vi "Teleop - Copy.vi"(10 "Match Info":T3={"Autonomous Elapsed Seconds"=0.0, "TeleOp Elapsed Seconds"=0.0, "Disabled Elapsed Seconds"=0.0, "Visited Autonomous"=FALSE, "Visited TeleOp"=FALSE, "Visited Disabled"=FALSE, "Autonomous Settings"={"Autonomous Style"=enum."Independent", "VI Refnum"=refnum}}, 11 "Call Context":T4) -> ()   [LabVIEW 2015]
doc: "This VI is called for each TeleOp packet received from the DS where the robot is not disabled. It is often used to read from the joysticks and update I/O or to update setpoints for timed control loops. It should complete and return within 20 milliseconds or it may miss DS packets."
uses:
  <vilib>/Rock Robotics/WPI/DriverStation/WPI_DriverStationDerivedRobotMode.ctl
  <vilib>/Rock Robotics/WPI/DriverStation/WPI_DriverStationMatch Info.ctl
  <vilib>/Rock Robotics/WPI/Joystick/WPI_JoystickDevRef.ctl
  <vilib>/Rock Robotics/WPI/Joystick/WPI_JoystickDeviceEnum.ctl
  <vilib>/Rock Robotics/WPI/Utilities/WPI_GetSetVariantRefNum.vi
  <vilib>/Rock Robotics/Network Tables/NT Read Boolean.vi
  <vilib>/Rock Robotics/Network Tables/NT Read Number.vi
  Robot Global Data.vi
  <vilib>/Rock Robotics/Network Tables/NT Write Numeric Array.vi
  <vilib>/Rock Robotics/Network Tables/NT Write Boolean Array.vi
  <vilib>/Rock Robotics/Network Tables/NT Write Number.vi
panel:
  in  "Intake Speed 2":dbl=-30.0 format="%#_13g"
  out "Joystick0":T1={"Device"=enum."USB 1"}
  out "Position Control":dbl
  in  "Intake Speed":dbl=-30.0 format="%#_13g"
  out "Sample Slider 0":dbl(slide) scale=0.0..5.0
  out "Sample Boolean 1":bool
  out "Sample Boolean 0":bool
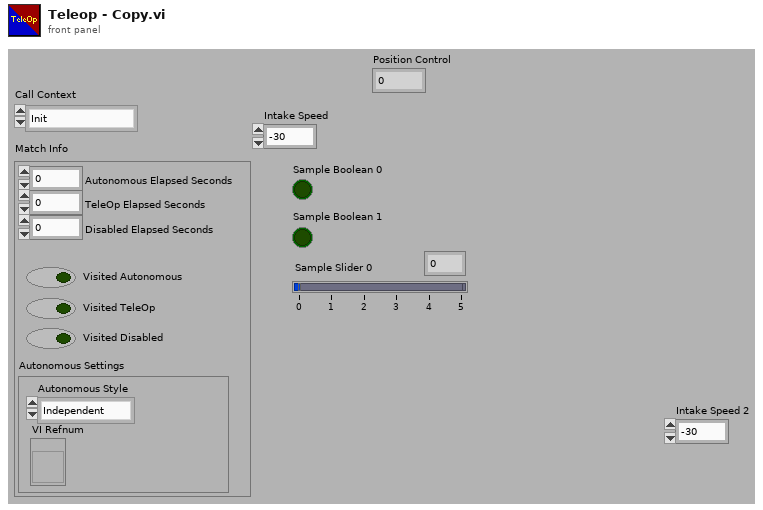
[diagram p1: front panel]
types:
  T1 = typedef "WPI_JoystickDevRef.ctl" = cluster{"Device":T2}
  T2 = typedef "WPI_JoystickDeviceEnum.ctl" = enum16{"USB 0", "USB 1", "USB 2", "USB 3", "USB 4", "USB 5"}
  T3 = typedef "WPI_DriverStationMatch Info.ctl" = cluster{"Autonomous Elapsed Seconds":dbl, "TeleOp Elapsed Seconds":dbl, "Disabled Elapsed Seconds":dbl, "Visited Autonomous":bool, "Visited TeleOp":bool, "Visited Disabled":bool, "Autonomous Settings":cluster{"Autonomous Style":enum16{"Iterative", "Independent"}, "VI Refnum":refnum<vi>}}
  T4 = typedef "WPI_DriverStationDerivedRobotMode.ctl" = enum16{"Init", "Execute", "Stop"}
  T5 = typedef "WPI_DigitalInputDevRef.ctl" = cluster{"DevStatus":errorcluster, "DIO Channel":T6}
  T6 = typedef "FPGA_DIOChannel.ctl" = enum8{"DIO 0", "DIO 1", "DIO 2", "DIO 3", "DIO 4", "DIO 5", "DIO 6", "DIO 7", "DIO 8", "DIO 9", "DIO MXP 0", "DIO MXP 1", "DIO MXP 2", "DIO MXP 3", "DIO MXP 4", "DIO MXP 5", "DIO MXP 6", "DIO MXP 7", "DIO MXP 8", "DIO MXP 9", "DIO MXP 10", "DIO MXP 11", "DIO MXP 12", "DIO MXP 13", "DIO MXP 14", "DIO MXP 15", "Invalid"}
  T7 = cluster{"LeftX":dbl, "LeftY":dbl, "LTrigger":dbl, "RTrigger":dbl, "RightX":dbl, "RightY":dbl, "RightY 2":dbl, "RightX 2":dbl}
  T8 = cluster{"ButtonA":bool, "ButtonB":bool, "ButtonX":bool, "ButtonY":bool, "ButtonLB":bool, "ButtonRB":bool, "ButtonBack":bool, "ButtonStart":bool, "Button1":bool, "Button2":bool}
  T9 = typedef "WPI_MotorControlDeviceRef.ctl" = cluster{"DeviceStatus":errorcluster, "Type":T10, "PWM":cluster{"PWM Channel":T11, "DeadBand":T12}, "CAN":cluster{"Device Number":u8, "Control Mode":T13, "Semaphore":T14, "Max Vout":dbl, "TalonSRX Control Mode":T15}, "Invert":bool}
  T10 = typedef "WPI_MotorControlType.ctl" = enum16{"PWM", "CAN", "CANTalonSRX"}
  T11 = typedef "FPGA_DIOPWMChannel.ctl" = enum8{"PWM 0", "PWM 1", "PWM 2", "PWM 3", "PWM 4", "PWM 5", "PWM 6", "PWM 7", "PWM 8", "PWM 9", "PWM MXP 0", "PWM MXP 1", "PWM MXP 2", "PWM MXP 3", "PWM MXP 4", "PWM MXP 5", "PWM MXP 6", "PWM MXP 7", "PWM MXP 8", "PWM MXP 9", "Invalid"}
  T12 = typedef "WPI_PWMDeadband.ctl" = cluster{"Name":string, "maxPositivePwm":i32, "minPositivePwm":i32, "centerPwm":i32, "maxNegativePwm":i32, "minNegativePwm":i32, "angularRange":u16}
  T13 = typedef "WPI_CANJaguar_ControlMode.ctl" = enum8{"Percent VBus", "Current", "Speed", "Position", "Voltage"}
  T14 = typedef "Semaphore RefNum" = refnum<k1>
  T15 = typedef "WPI_CANTalonSRX_APIControlMode.ctl" = enum8{"Percent VBus", "Speed", "Position", "Slave", "Unchanged / Invalid", "Voltage Compensation", "Current", "Motion Profile"}
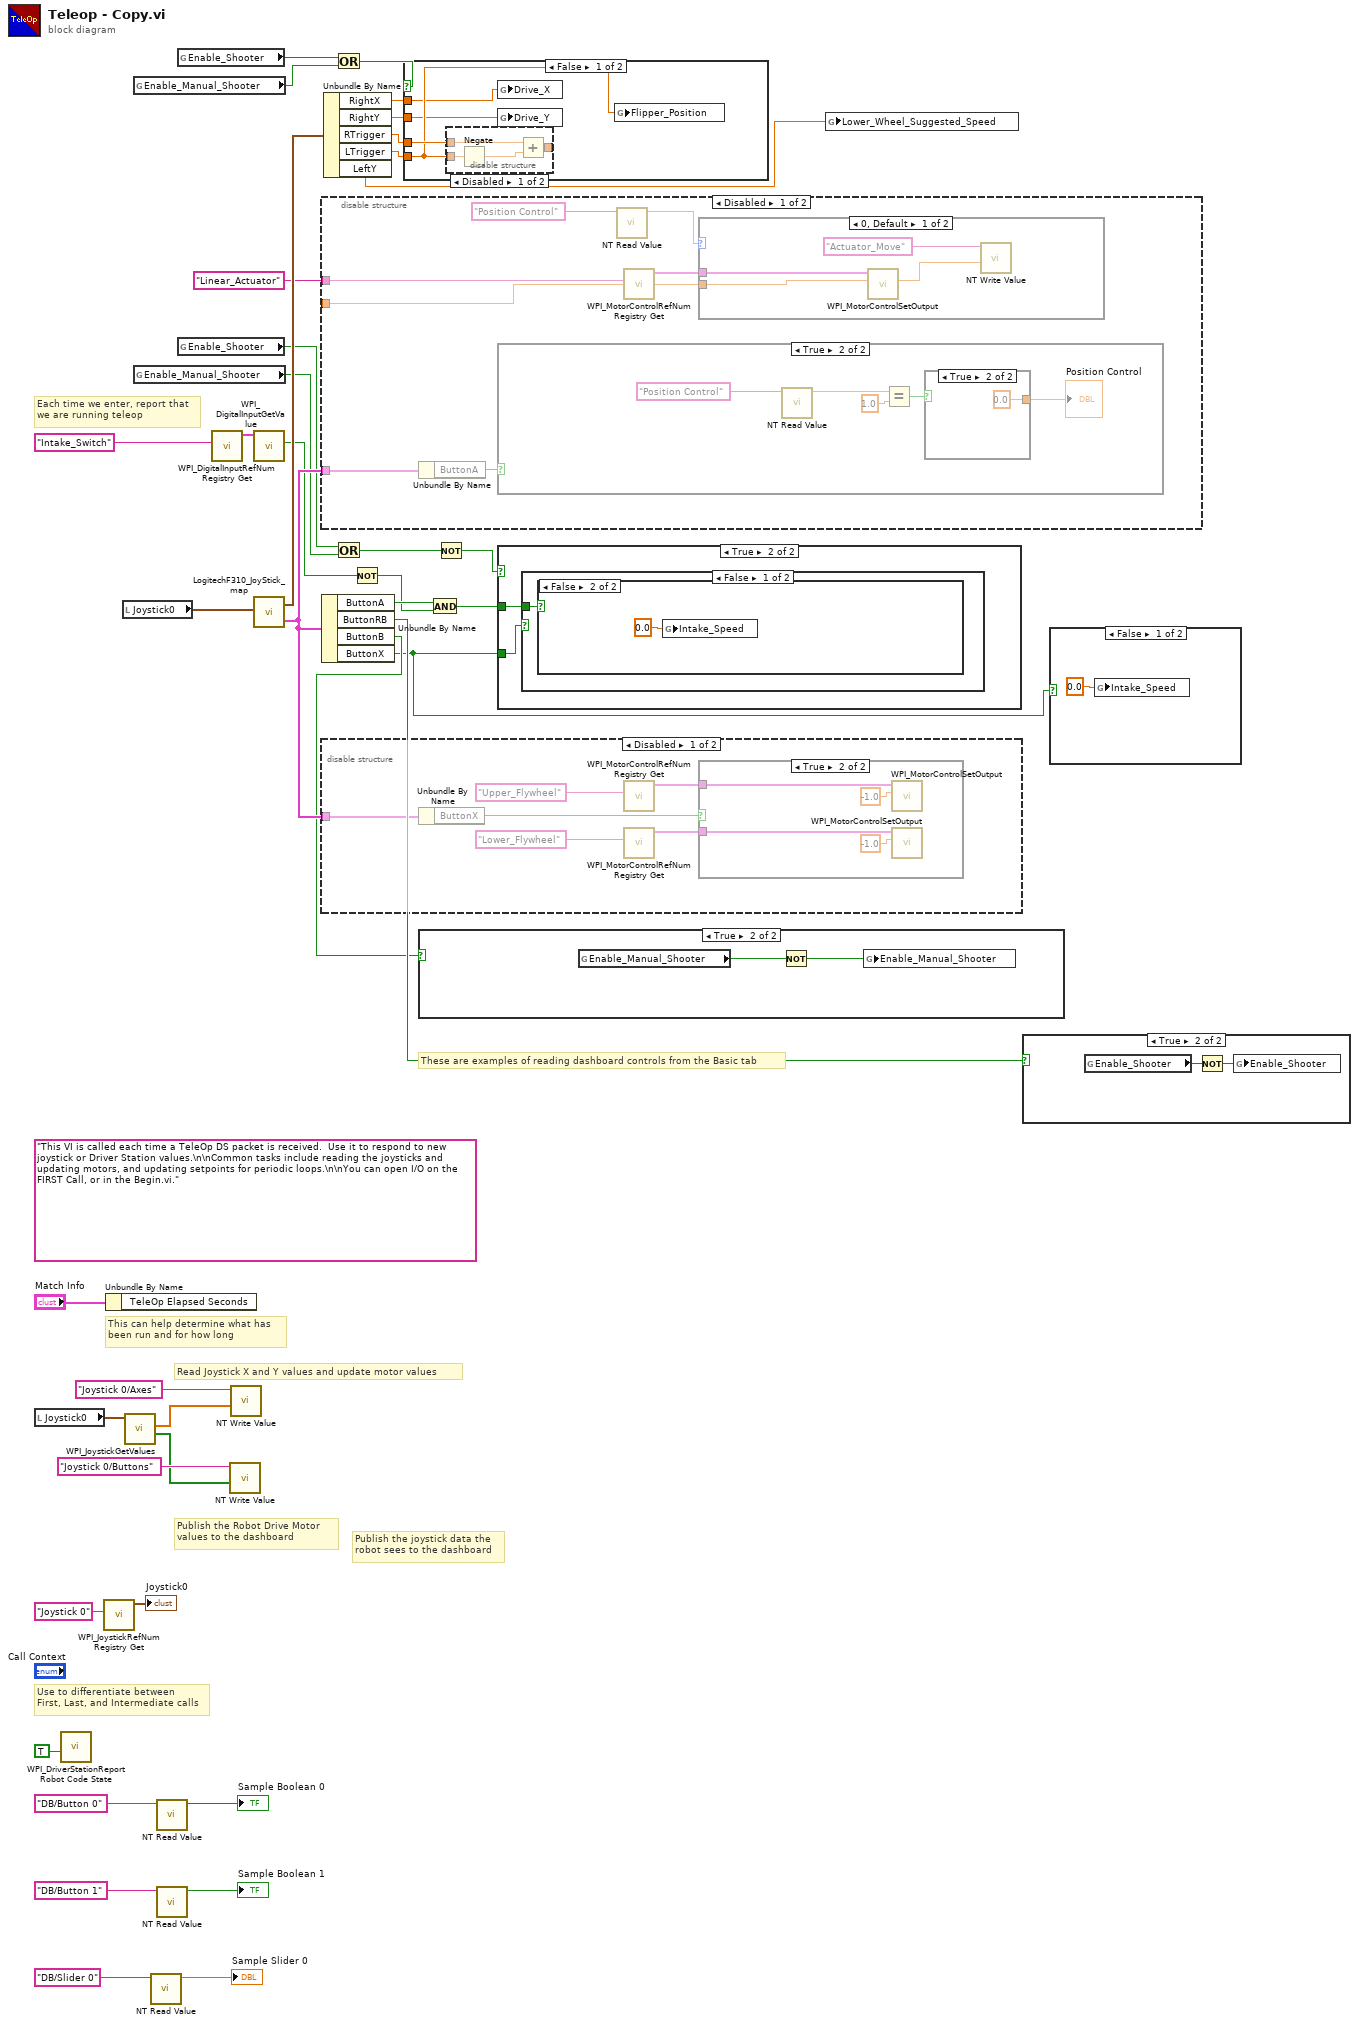
[diagram p0: block diagram]
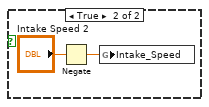
[diagram p2: hidden frame]
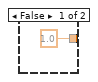
[diagram p6: hidden frame]
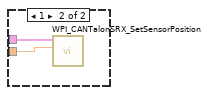
[diagram p7: hidden frame]
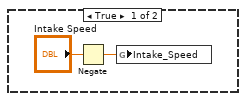
[diagram p10: hidden frame]
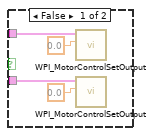
[diagram p14: hidden frame]
diagram:
  (unwired) "This VI is called each time a TeleOp DS packet is received.  Use it to respond to new joystick or Driver Station values.\n\nCommon tasks include reading the joysticks and updating motors, and updating setpoints for periodic loops.\n\nYou can open I/O on the FIRST Call, or in the Begin.vi."
  # "These are examples of reading dashboard controls from the Basic tab"
  # "Publish the Robot Drive Motor\nvalues to the dashboard"
  # "Publish the joystick data the\nrobot sees to the dashboard"
  # "Each time we enter, report that\nwe are running teleop"
  # "Use to differentiate between\nFirst, Last, and Intermediate calls"
  # "This can help determine what has\nbeen run and for how long"
  # "Read Joystick X and Y values and update motor values"
  n1 = local read "Joystick0"() -> (w8:T1)
  n2 = call <vilib>:"WPI_DriverStationReport Robot Code State.vi"("TeleOp"=TRUE ("Autonomous")) -> ()  [unwired: 10 in, 1 out]
  n3 = call <vilib>:"WPI_JoystickRefNum Registry Get.vi"("refnum name"="Joystick 0") -> ("JoystickDevRef"=→"Joystick0":T1)  [unwired: 1 in, 9 out]
  n4 = Unbundle By Name("Match Info") -> ()  [unwired: 1 out]
  n5 = local read "Joystick0"() -> (w5:T1)
  n6 = call <vilib>:"WPI_JoystickGetValues.vi"("JoystickDevRef"=w8) -> ("Buttons"=w34:bool[], "Axes"=w35:dbl[])  [unwired: 6 in, 3 out]
  n7 = global read "Robot Global Data.vi" "Enable_Manual_Shooter"() -> (w11:bool)
  n8 = global read "Robot Global Data.vi" "Enable_Manual_Shooter"() -> (w13:bool)
  n9 = call-poly <vilib>:"NT Read Value.vi"("Name"="DB/Slider 0" ("refnum name")) -> ("Numeric"=→"Sample Slider 0":dbl)  [unwired: 9 in, 1 out]
  n10 = call-poly <vilib>:"NT Read Value.vi"("Name"="DB/Button 0" ("refnum name")) -> ("Boolean"=→"Sample Boolean 0":bool)  [unwired: 9 in, 1 out]
  n11 = call-poly <vilib>:"NT Read Value.vi"("Name"="DB/Button 1" ("refnum name")) -> ("Boolean"=→"Sample Boolean 1":bool)  [unwired: 9 in, 1 out]
  n12 = global read "Robot Global Data.vi" "Enable_Shooter"() -> (w19:bool)
  n13 = global read "Robot Global Data.vi" "Enable_Shooter"() -> (w18:bool)
  n14 = call <vilib>:"WPI_DigitalInputRefNum Registry Get.vi"("refnum name"="Intake_Switch") -> ("DigitalInputDevRef"=w23:T5)  [unwired: 9 in, 1 out]
  n15 = call-poly <vilib>:"NT Write Value.vi"("Boolean Array"=w34, "Name"="Joystick 0/Buttons") -> ()  [unwired: 9 in, 1 out]
  n16 = call-poly <vilib>:"NT Write Value.vi"("Numeric Array"=w35, "Name"="Joystick 0/Axes") -> ()  [unwired: 9 in, 1 out]
  n17 = call <vilib>:"WPI_DigitalInputGetValue.vi"("DigitalInputDevRef"=w23) -> ("Value"=w3:bool)  [unwired: 8 in, 2 out]
  n18 = call "LogitechF310_JoyStick_map.vi"("JoystickDevRef"=w5) -> ("AxesCluster"=w27:T7, "ButtonsCluster"=w24:T8)
  n19 = disable-structure shown="Disabled" {
    disable-tunnel: "Linear_Actuator" ("refnum name") -> [w47 _]
    disable-tunnel: _ -> [w45 _]
    disable-tunnel: w24 -> [w44 _]
    frame Disabled {
      n20 = Unbundle By Name(w44) -> ("ButtonA"=w43:bool)
      n21 = case shown="True" w43 {
        frame False {
        }
        frame True {
          n22 = call-poly <vilib>:"NT Read Value.vi"("Name"="Position Control") -> ("Numeric"=w49:dbl)  [unwired: 9 in, 1 out]
          n23 = Equal?(x=w49, y=1.0) -> (x = y?=w51:bool)
          n24 = case shown="True" w51 {
            tunnel: [1.0 ("Position Control") 0.0 ("Position Control")] -> w48
            frame False {
            }
            frame True {
            }
          }
          "Position Control" <- w48
        }
      }
      n25 = call-poly <vilib>:"NT Read Value.vi"("Name"="Position Control") -> ("Numeric"=w41:dbl)  [unwired: 9 in, 1 out]
      n26 = call <vilib>:"WPI_MotorControlRefNum Registry Get.vi"("refnum name"=w47) -> ("MotorControlDevRef"=w46:T9)  [unwired: 9 in, 1 out]
      n27 = case shown="0, Default" w41 {
        tunnel: w46 -> [w55 w60]
        tunnel: w45 -> [w56 w59]
        frame 0, Default {
          n28 = call <vilib>:"WPI_MotorControlSetOutput.vi"("Output"=w56, "MotorControlDevRef"=w55) -> ("Motor Output"=w58:dbl)  [unwired: 7 in, 2 out]
          n29 = call-poly <vilib>:"NT Write Value.vi"("Numeric"=w58, "Name"="Actuator_Move") -> ()  [unwired: 9 in, 1 out]
        }
        frame 1 {
          n30 = call <vilib>:"WPI_CANTalonSRX_SetSensorPosition.vi"("New Sensor Position"=w59, "CAN Talon SRX Ref"=w60) -> ()  [unwired: 8 in, 2 out]
        }
      }
    }
    frame Enabled {
    }
  }
  n31 = Unbundle By Name(w24) -> ("ButtonA"=w22:bool, "ButtonRB"=w16:bool, "ButtonB"=w15:bool, "ButtonX"=w1:bool)
  n32 = disable-structure shown="Disabled" {
    disable-tunnel: w24 -> [w61 _]
    frame Disabled {
      n33 = Unbundle By Name(w61) -> ("ButtonX"=w66:bool)
      n34 = call <vilib>:"WPI_MotorControlRefNum Registry Get.vi"("refnum name"="Upper_Flywheel") -> ("MotorControlDevRef"=w63:T9)  [unwired: 9 in, 1 out]
      n35 = call <vilib>:"WPI_MotorControlRefNum Registry Get.vi"("refnum name"="Lower_Flywheel") -> ("MotorControlDevRef"=w62:T9)  [unwired: 9 in, 1 out]
      n36 = case shown="True" w66 {
        tunnel: w63 -> [w69 w74]
        tunnel: w62 -> [w70 w73]
        frame False {
          n37 = call <vilib>:"WPI_MotorControlSetOutput.vi"("Output"=0.0, "MotorControlDevRef"=w69) -> ()  [unwired: 7 in, 3 out]
          n38 = call <vilib>:"WPI_MotorControlSetOutput.vi"("Output"=0.0, "MotorControlDevRef"=w70) -> ()  [unwired: 7 in, 3 out]
        }
        frame True {
          n39 = call <vilib>:"WPI_MotorControlSetOutput.vi"("Output"=-1.0, "MotorControlDevRef"=w74) -> ()  [unwired: 7 in, 3 out]
          n40 = call <vilib>:"WPI_MotorControlSetOutput.vi"("Output"=-1.0, "MotorControlDevRef"=w73) -> ()  [unwired: 7 in, 3 out]
        }
      }
    }
    frame Enabled {
    }
  }
  n41 = Unbundle By Name(w27) -> ("RightX"=w21:dbl, "RightY"=w20:dbl, "RTrigger"=w7:dbl, "LTrigger"=w6:dbl, "LeftY"=w4:dbl)
  n42 = Or(x=w19, y=w11) -> (x .or. y?=w12:bool)
  n43 = Or(x=w18, y=w13) -> (x .or. y?=w14:bool)
  n44 = Not(x=w3) -> (.not. x?=w2:bool)
  n45 = case shown="False" w12 {
    tunnel: w21 -> [w76 _]
    tunnel: w20 -> [w75 _]
    tunnel: w7 -> [w78 _]
    tunnel: w6 -> [w77 _]
    frame False {
      n46 = disable-structure shown="Disabled" {
        disable-tunnel: [w81 _] -> _
        disable-tunnel: w78 -> [w80 _]
        disable-tunnel: w77 -> [w79 _]
        frame Disabled {
          n47 = Negate(x=w79) -> (-x=w82:dbl)
          n48 = Add(x=w80, y=w82) -> (x+y=w81:dbl)
        }
        frame Enabled {
        }
      }
      n49 = global write "Robot Global Data.vi" "Drive_X"(w76) -> ()
      n50 = global write "Robot Global Data.vi" "Drive_Y"(w75) -> ()
      n51 = global write "Robot Global Data.vi" "Flipper_Position"(w77) -> ()
    }
    frame True {
    }
  }
  n52 = case shown="True" w15 {
    frame False {
    }
    frame True {
      n53 = global read "Robot Global Data.vi" "Enable_Manual_Shooter"() -> (w84:bool)
      n54 = Not(x=w84) -> (.not. x?=w83:bool)
      n55 = global write "Robot Global Data.vi" "Enable_Manual_Shooter"(w83) -> ()
    }
  }
  n56 = And(x=w22, y=w2) -> (x .and. y?=w10:bool)
  n57 = Not(x=w14) -> (.not. x?=w17:bool)
  n58 = case shown="True" w17 {
    tunnel: w10 -> [_ w86]
    tunnel: w1 -> [_ w85]
    frame False {
    }
    frame True {
      n59 = case shown="False" w85 {
        tunnel: w86 -> [w87 _]
        frame False {
          n60 = case shown="False" w87 {
            frame True {
              n61 = Negate(x="Intake Speed") -> (-x=w88:dbl)
              n62 = global write "Robot Global Data.vi" "Intake_Speed"(w88) -> ()
            }
            frame False {
              n63 = global write "Robot Global Data.vi" "Intake_Speed"(0.0 ("Output")) -> ()
            }
          }
        }
        frame True {
        }
      }
    }
  }
  n64 = global write "Robot Global Data.vi" "Lower_Wheel_Suggested_Speed"(w4) -> ()
  n65 = case shown="True" w16 {
    frame False {
    }
    frame True {
      n66 = global read "Robot Global Data.vi" "Enable_Shooter"() -> (w92:bool)
      n67 = Not(x=w92) -> (.not. x?=w91:bool)
      n68 = global write "Robot Global Data.vi" "Enable_Shooter"(w91) -> ()
    }
  }
  n69 = case shown="False" w1 {
    frame False {
      n70 = global write "Robot Global Data.vi" "Intake_Speed"(0.0 ("Output")) -> ()
    }
    frame True {
      n71 = Negate(x="Intake Speed 2") -> (-x=w94:dbl)
      n72 = global write "Robot Global Data.vi" "Intake_Speed"(w94) -> ()
    }
  }
